vi "Get NT PID Parameter.vi"(1 "NT Path":string) -> (0 "PID Gains":T1)   [LabVIEW 2015]
uses:
  <vilib>/Rock Robotics/Network Tables/NT Read Number.vi
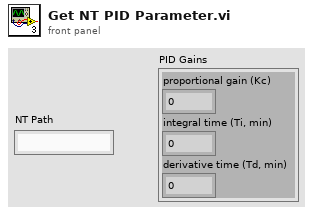
[diagram p1: front panel]
types:
  T1 = cluster{"proportional gain (Kc)":dbl, "integral time (Ti, min)":dbl, "derivative time (Td, min)":dbl}
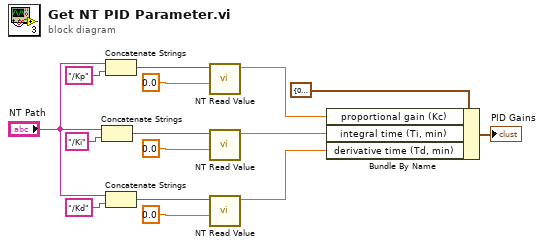
[diagram p0: block diagram]
diagram:
  n1 = Concatenate Strings("NT Path", "/Ki" ("string")) -> (w2:string)
  n2 = Concatenate Strings("NT Path", "/Kp" ("string")) -> (w3:string)
  n3 = Concatenate Strings("NT Path", "/Kd" ("string")) -> (w1:string)
  n4 = call-poly <vilib>:"NT Read Value.vi"("Default Value"=0.0, "Name"=w3) -> ("Numeric"=w10:dbl)  [unwired: 8 in, 1 out]
  n5 = call-poly <vilib>:"NT Read Value.vi"("Default Value"=0.0, "Name"=w2) -> ("Numeric"=w11:dbl)  [unwired: 8 in, 1 out]
  n6 = call-poly <vilib>:"NT Read Value.vi"("Default Value"=0.0, "Name"=w1) -> ("Numeric"=w12:dbl)  [unwired: 8 in, 1 out]
  n7 = Bundle By Name(cluster=T1 {"proportional gain (Kc)"=0.0, "integral time (Ti, min)"=0.0, "derivative time (Td, min)"=0.0} ("Arm Parameters.PID gains"), "proportional gain (Kc)"=w10, "integral time (Ti, min)"=w11, "derivative time (Td, min)"=w12) -> (→"PID Gains":T1)
